vi "Read Cal Standard Port.vi"(8 "error in (no error)":errorcluster, 11 "Vector Path in":refnum<class "Vector Abstract Path.lvclass">) -> (0 "error out":errorcluster, 2 "Cal Standard Port":string, 3 "Vector Path out":refnum<class "Vector Abstract Path.lvclass">)   [LabVIEW 2023, in "RFFixtureCharact.Public.lvlib" / "Vector Abstract Path.lvclass"]
uses:
  Vector Abstract Path.lvclass
  Vector Abstract Path.lvclass/Vector Abstract Path.ctl
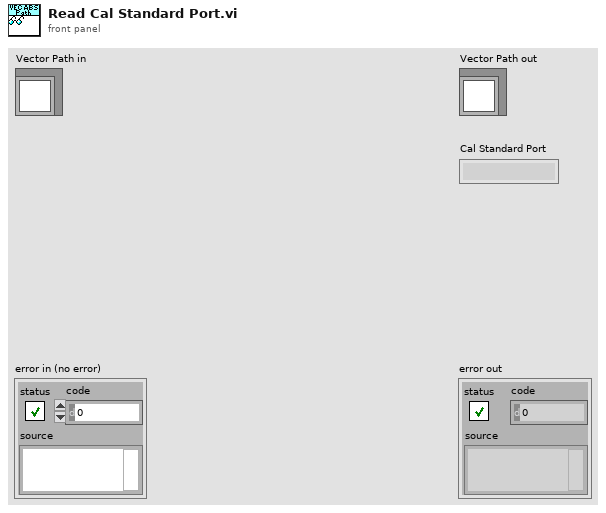
[diagram p1: front panel]
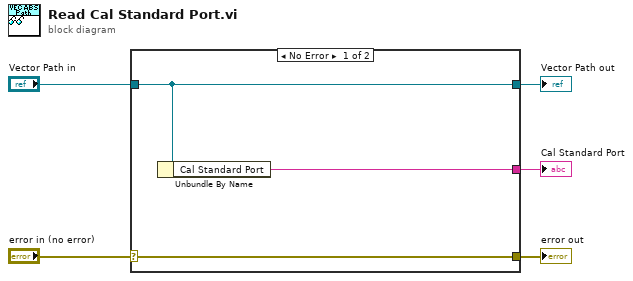
[diagram p0: block diagram]
diagram:
  n1 = case shown="No Error" "error in (no error)" {
    selector: "error in (no error)" -> [w8 w9]
    tunnel: [w8 w9] -> w4
    tunnel: [w7 w10] -> w2
    tunnel: "Vector Path in" -> [w7 w10]
    tunnel: [w6 _] -> w1
    frame No Error {
      n2 = Unbundle By Name(w7) -> ("Cal Standard Port"=w6:string)
    }
    frame Error {
    }
  }
  "error out" <- w4
  "Vector Path out" <- w2
  "Cal Standard Port" <- w1
